vi "Sensor_data_to_value_step2_convert.vi"(5 "Graph format (T)":bool=TRUE, 10 "Sensor data resolved sign":i32, 11 "Sensor type":u8 format="%x") -> (2 "Signal legend":string, 3 "Value ouptut":dbl)   [LabVIEW 2013]
doc: "Converts sensor type data to human readable value format\nADC to mV\nLight sensor to Lux\nTemperature to [10*degC]\nRelative humidity to [10*%RH]\nNDIR module data to ACT/DIV gas value [x/1000] (to get real ratio, divide by 1000)\nNDIR module temperature to [10*degC]\n\nGraph format \n(T) - will format values so it can be displayed better on graph. Analog Ins are in mV (not volts). T and RH is deg C *10 and RH*10\n(F) - will change format to Votls and degC and RH. Marked appropriately in legend string.\n\nAlso determines if sensor raw data are signed or unsigned. Output sensor data int32 will give correct result."
panel:
  # "Converts sensor type data to human readable value format\nADC to mV\nLight sensor to Lux\nTemperature to [10*degC]\nRelative humidity to [10*%RH]"
  # "Detailed (F)"
  # "As in graphs(T)"
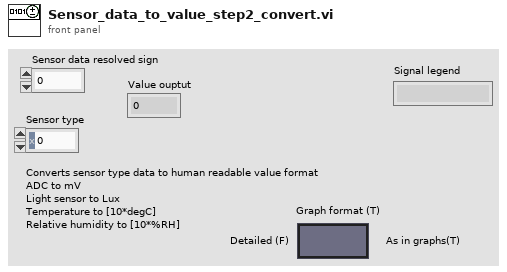
[diagram p1: front panel]
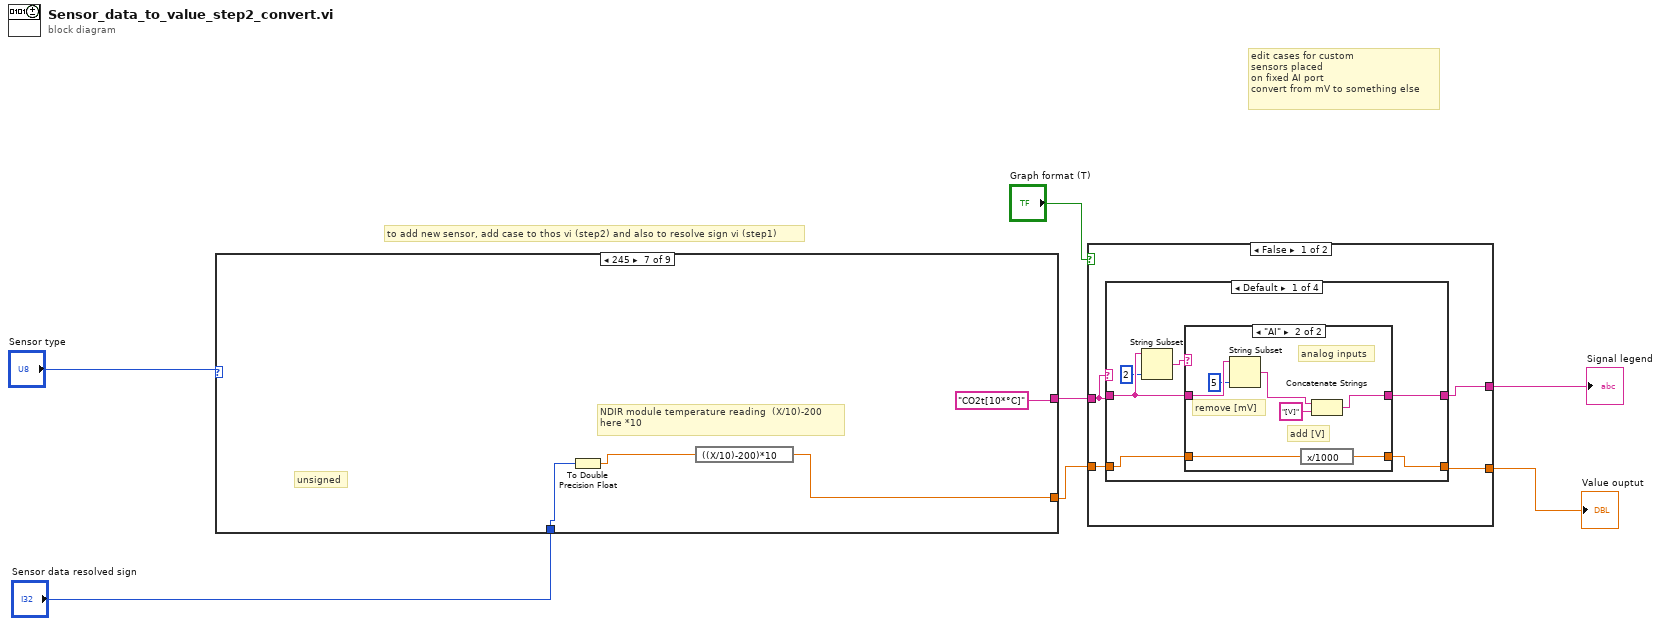
[diagram p0: block diagram]
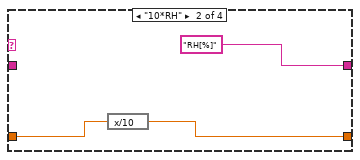
[diagram p3: hidden frame]
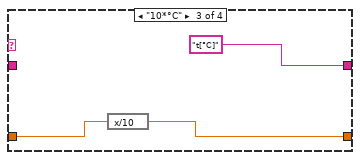
[diagram p4: hidden frame]
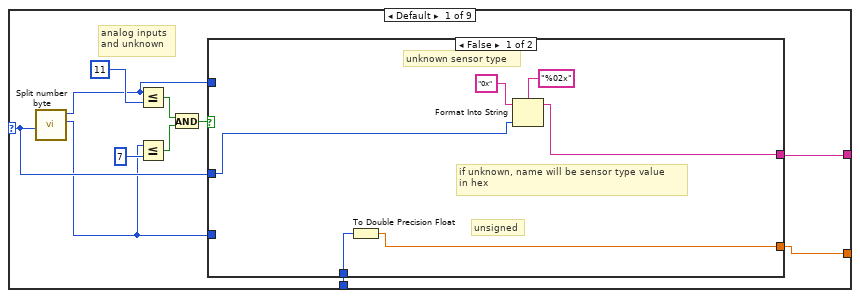
[diagram p7: hidden frame]
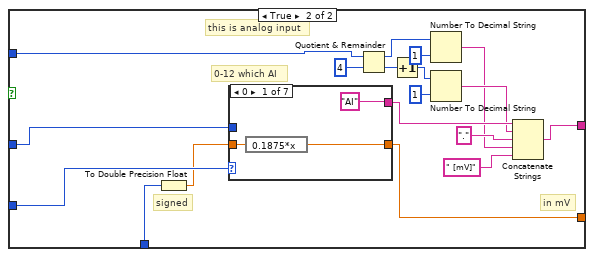
[diagram p8: hidden frame]
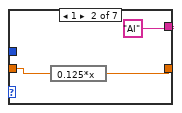
[diagram p9: hidden frame]
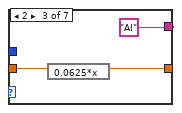
[diagram p10: hidden frame]
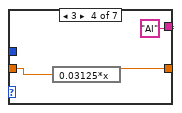
[diagram p11: hidden frame]
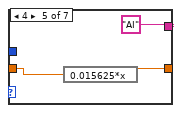
[diagram p12: hidden frame]
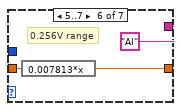
[diagram p13: hidden frame]
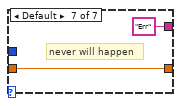
[diagram p14: hidden frame]
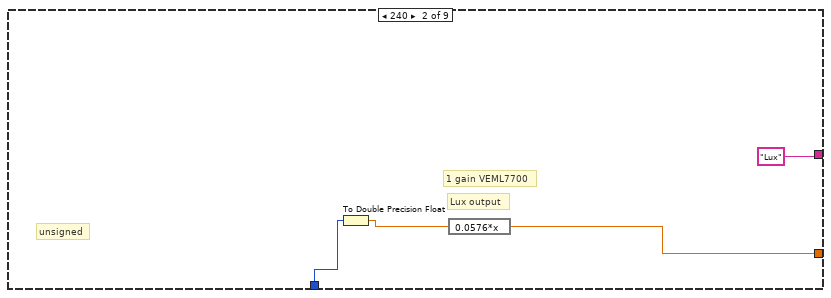
[diagram p15: hidden frame]
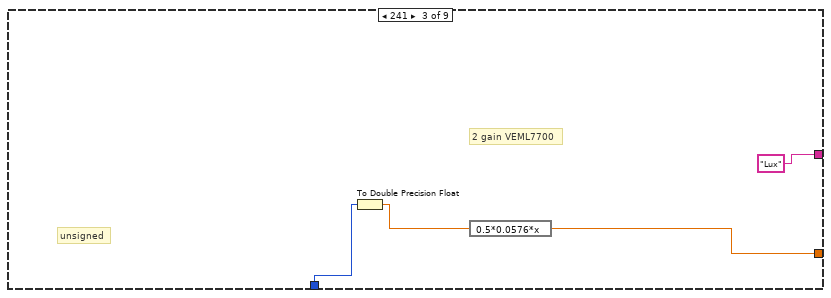
[diagram p16: hidden frame]
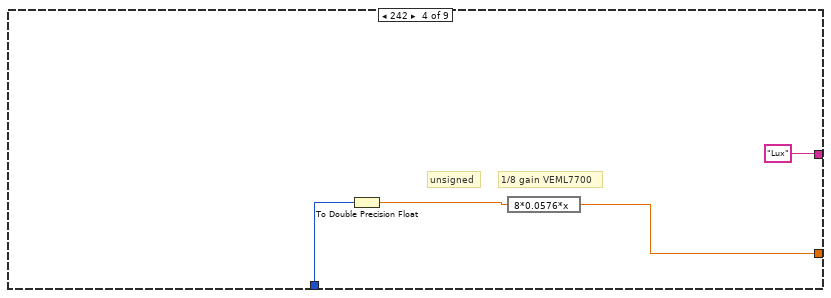
[diagram p17: hidden frame]
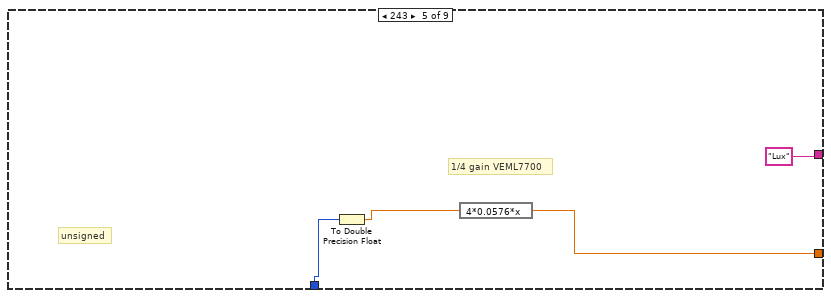
[diagram p18: hidden frame]
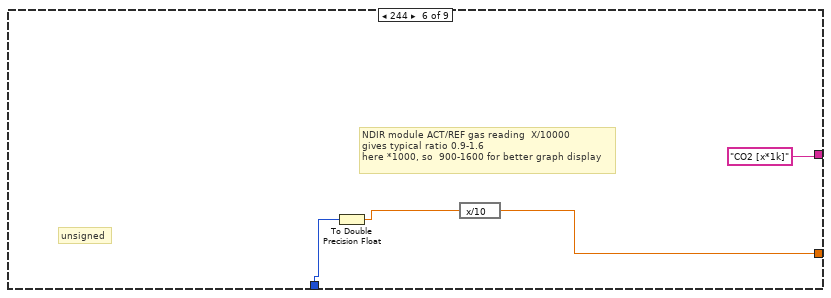
[diagram p19: hidden frame]
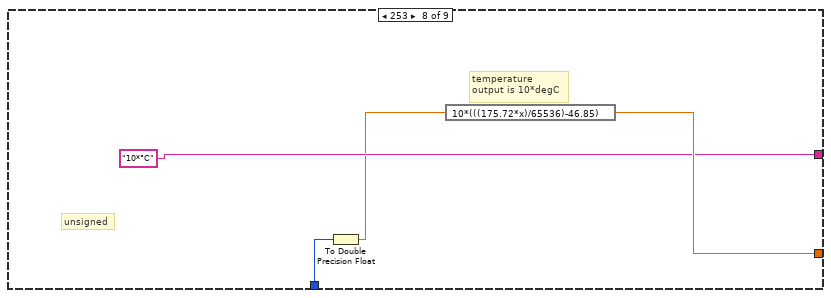
[diagram p20: hidden frame]
diagram:
  # "to add new sensor, add case to thos vi (step2) and also to resolve sign vi (step1)"
  # "edit cases for custom \nsensors placed\non fixed AI port\nconvert from mV to something else"
  n1 = case shown="245" "Sensor type" {
    selector: "Sensor type" -> [w11 _ _ _ _ _ _ _ _]
    tunnel: [w12 w66 w70 w74 w78 w82 w86 w90 w94] -> w7
    tunnel: [w13 "Lux" ("initial string") "Lux" ("initial string") "Lux" ("initial string") "Lux" ("initial string") "CO2 [x*1k]" ("initial string") "CO2t[10*°C]" ("initial string") "10*°C" ("initial string") "10*RH" ("initial string")] -> w4
    tunnel: "Sensor data resolved sign" -> [w8 w64 w68 w72 w76 w80 w84 w88 w92]
    frame Default {
      # "analog inputs\nand unknown"
      n2 = call "Split number byte.vi"("x"=w11) -> ("lo(x)"=w10:u8, "hi(x)"=w9:u8)  [unwired: 9 in]
      n3 = Less Or Equal?(x=w9, y=u8 11) -> (x <= y?=w16:bool)
      n4 = Less Or Equal?(x=w10, y=u8 7) -> (x <= y?=w15:bool)
      n5 = And(x=w16, y=w15) -> (x .and. y?=w14:bool)
      n6 = case shown="False" w14 {
        tunnel: w10 -> [_ w42]
        tunnel: w11 -> [w22 w41]
        tunnel: [w21 w34] -> w13
        tunnel: [w19 w33] -> w12
        tunnel: w9 -> [_ w29]
        tunnel: w8 -> [w20 w26]
        frame False {
          # "unsigned"
          # "if unknown, name will be sensor type value\nin hex"
          # "unknown sensor type"
          n7 = To Double Precision Float(number=w20) -> (double precision float=w19:dbl)
          n8 = Format Into String(format string="%02x", initial string="0x", w22) -> (resulting string=w21:string)  [unwired: 1 in, 1 out]
        }
        frame True {
          # "in mV"
          # "signed"
          # "0-12 which AI"
          # "this is analog input"
          n9 = To Double Precision Float(number=w26) -> (double precision float=w27:dbl)
          n10 = case shown="0" w42 {
            tunnel: [w45 w48 w51 w54 w57 w60 w62] -> w33
            tunnel: ["AI" ("initial string") "AI" ("initial string") "AI" ("initial string") "AI" ("initial string") "AI" ("initial string") "AI" ("initial string") "Err" ("initial string")] -> w36
            tunnel: w27 -> [w43 w46 w49 w52 w55 w58 w62]
            tunnel: w41 -> [_ _ _ _ _ _ _]
            frame 0 {
              n11 = expression code="0.1875*x"(w43) -> (w45:dbl)
            }
            frame 1 {
              n12 = expression code="0.125*x"(w46) -> (w48:dbl)
            }
            frame 2 {
              n13 = expression code="0.0625*x"(w49) -> (w51:dbl)
            }
            frame 3 {
              n14 = expression code="0.03125*x"(w52) -> (w54:dbl)
            }
            frame 4 {
              n15 = expression code="0.015625*x"(w55) -> (w57:dbl)
            }
            frame 5..7 {
              # "0.256V range"
              n16 = expression code="0.007813*x"(w58) -> (w60:dbl)
            }
            frame Default {
              # "never will happen"
            }
          }
          n17 = Quotient & Remainder(x=w29, y=u8 4) -> (x-y*floor(x/y)=w30:u8, floor(x/y)=w39:u8)
          n18 = Increment(x=w39) -> (x+1=w28:u8)
          n19 = Number To Decimal String(number=w30, width (-)=i16 1) -> (decimal integer string=w31:string)
          n20 = Number To Decimal String(number=w28, width (-)=i16 1) -> (decimal integer string=w32:string)
          n21 = Concatenate Strings(w36, w32, "." ("string"), w31, " [mV]" ("string")) -> (w34:string)
        }
      }
    }
    frame 240 {
      # "unsigned"
      # "Lux output"
      # "1 gain VEML7700"
      n22 = To Double Precision Float(number=w64) -> (double precision float=w63:dbl)
      n23 = expression code="0.0576*x"(w63) -> (w66:dbl)
    }
    frame 241 {
      # "unsigned"
      # "2 gain VEML7700"
      n24 = To Double Precision Float(number=w68) -> (double precision float=w67:dbl)
      n25 = expression code="0.5*0.0576*x"(w67) -> (w70:dbl)
    }
    frame 242 {
      # "unsigned"
      # "1/8 gain VEML7700"
      n26 = To Double Precision Float(number=w72) -> (double precision float=w71:dbl)
      n27 = expression code="8*0.0576*x"(w71) -> (w74:dbl)
    }
    frame 243 {
      # "unsigned"
      # "1/4 gain VEML7700"
      n28 = To Double Precision Float(number=w76) -> (double precision float=w75:dbl)
      n29 = expression code="4*0.0576*x"(w75) -> (w78:dbl)
    }
    frame 244 {
      # "unsigned"
      # "NDIR module ACT/REF gas reading\t\tX/10000\ngives typical ratio 0.9-1.6\nhere *1000, so  900-1600 for better graph display"
      n30 = To Double Precision Float(number=w80) -> (double precision float=w79:dbl)
      n31 = expression code="x/10"(w79) -> (w82:dbl)
    }
    frame 245 {
      # "unsigned"
      # "NDIR module temperature reading\t\t(X/10)-200\nhere *10"
      n32 = To Double Precision Float(number=w84) -> (double precision float=w83:dbl)
      n33 = expression code="((X/10)-200)*10"(w83) -> (w86:dbl)
    }
    frame 253 {
      # "unsigned"
      # "temperature\noutput is 10*degC"
      n34 = To Double Precision Float(number=w88) -> (double precision float=w87:dbl)
      n35 = expression code="10*(((175.72*x)/65536)-46.85)"(w87) -> (w90:dbl)
    }
    frame 254 {
      # "unsigned"
      # "RH\noutput is 10*%RH"
      n36 = To Double Precision Float(number=w92) -> (double precision float=w91:dbl)
      n37 = expression code="10*(((125*x)/65536)-6)"(w91) -> (w94:dbl)
    }
  }
  n38 = case shown="False" "Graph format (T)" {
    tunnel: w7 -> [w98 w122]
    tunnel: [w97 w122] -> w6
    tunnel: [w96 w123] -> w5
    tunnel: w4 -> [w95 w123]
    frame False {
      n39 = case shown="Default" w95 {
        tunnel: w98 -> [w103 w116 w119 w120]
        tunnel: [w102 w115 w118 w120] -> w97
        tunnel: [w104 "RH[%]" ("initial string") "t[°C]" ("initial string") w121] -> w96
        tunnel: w95 -> [w101 _ _ w121]
        frame Default {
          n40 = String Subset(string=w101, length (rest)=2 ("length (rest)")) -> (substring=w99:string)  [unwired: 1 in]
          n41 = case shown="\"AI\"" w99 {
            tunnel: [w105 w112] -> w104
            tunnel: w103 -> [w106 w111]
            tunnel: [w106 w110] -> w102
            tunnel: w101 -> [w105 w109]
            frame "False", Default {
            }
            frame "AI" {
              # "add [V]"
              # "remove [mV]"
              # "analog inputs"
              n42 = String Subset(string=w109, length (rest)=5 ("length (rest)")) -> (substring=w107:string)  [unwired: 1 in]
              n43 = expression code="x/1000"(w111) -> (w110:dbl)
              n44 = Concatenate Strings(w107, "[V]" ("string")) -> (w112:string)
            }
          }
        }
        frame "10*RH" {
          n45 = expression code="x/10"(w116) -> (w115:dbl)
        }
        frame "10*°C" {
          n46 = expression code="x/10"(w119) -> (w118:dbl)
        }
        frame "Lux" {
        }
      }
    }
    frame True {
    }
  }
  "Value ouptut" <- w6
  "Signal legend" <- w5
